vi "Th_stopwatch_TimeReset.vi"   [LabVIEW 2018]
uses:
  Th_GUI.vi
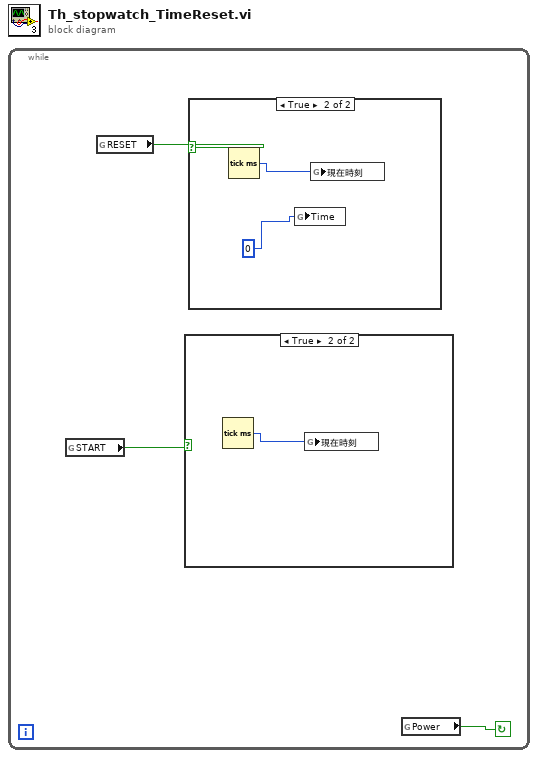
[diagram p0: block diagram]
diagram:
  n1 = while {
    stop <- w1 continue-if-true
    n2 = global read "Th_GUI.vi" "START"() -> (w2:bool)
    n3 = global read "Th_GUI.vi" "RESET"() -> (w3:bool)
    n4 = case shown="TRUE" w2 {
      frame False {
      }
      frame True {
        n5 = Tick Count (ms)() -> (millisecond timer value=w4:u32)
        n6 = global write "Th_GUI.vi" "現在時刻"(w4) -> ()
      }
    }
    n7 = case shown="TRUE" w3 {
      frame False {
      }
      frame True {
        n8 = Tick Count (ms)() -> (millisecond timer value=w5:u32)
        n9 = global write "Th_GUI.vi" "Time"(0) -> ()
        n10 = global write "Th_GUI.vi" "現在時刻"(w5) -> ()
      }
    }
    n11 = global read "Th_GUI.vi" "Power"() -> (w1:bool)
  }
